vi "超标留样启动流程.vi"   [LabVIEW 2016, in "DR803M4.lvlib"]
uses:
  DR803M4.lvlib
  Global variable/input variable.vi
types:
  T1 = cluster{"远程留样":u16, "门禁标志":u16, "门禁密码":u32, "采样器进程":u16, "版本号":string, "启停":u16, "当前瓶号":u16, "采样模式选择":u16, "单次采样量":u16, "时间间隔":u16}
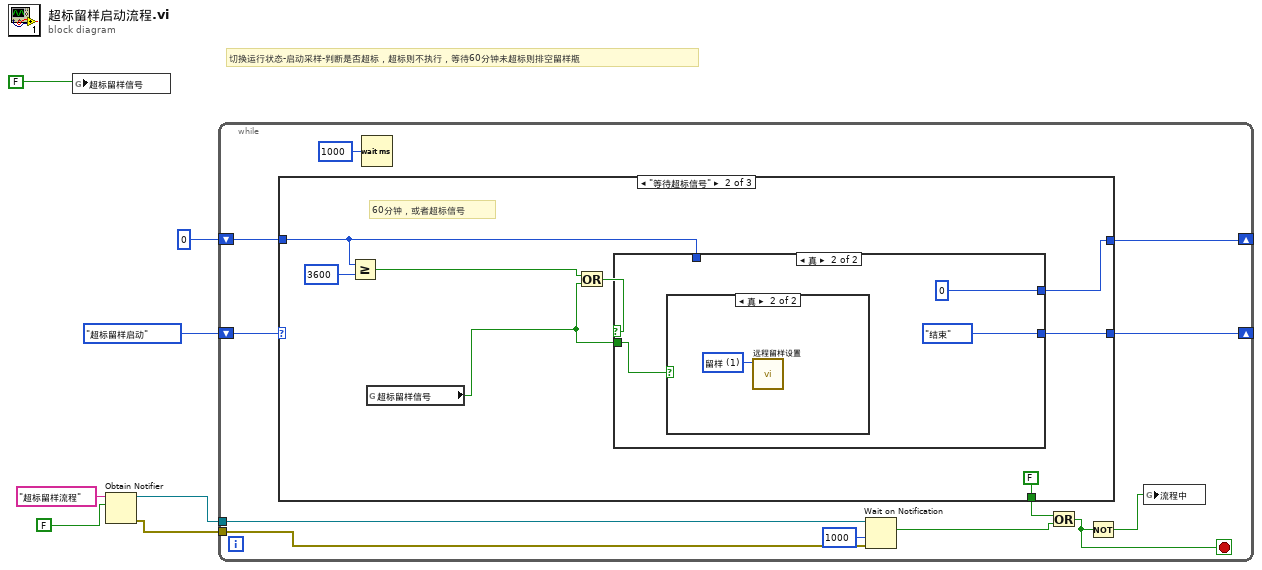
[diagram p0: block diagram]
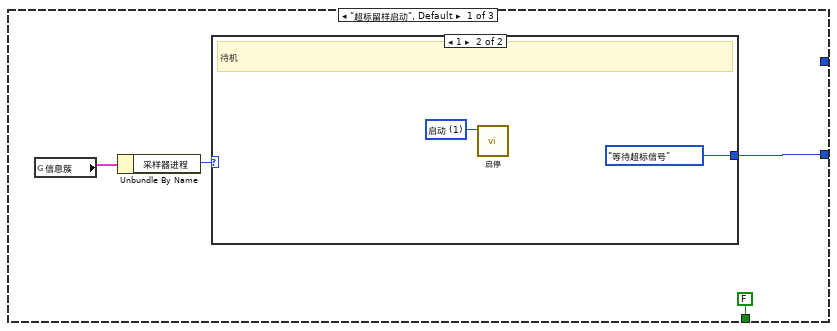
[diagram p2: hidden frame]
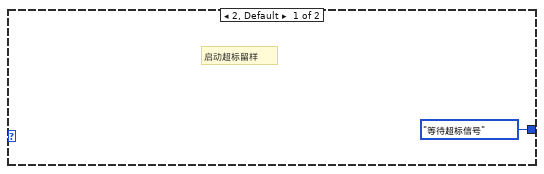
[diagram p3: hidden frame]
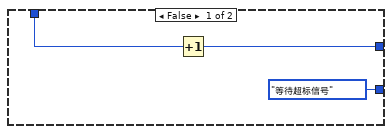
[diagram p4: hidden frame]
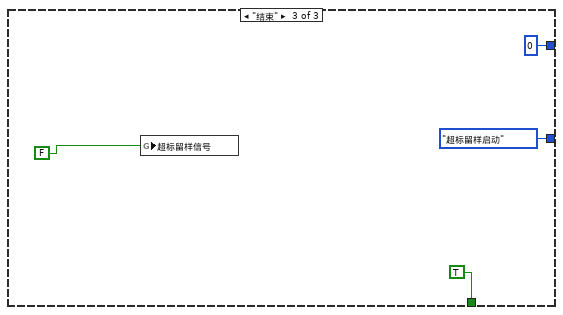
[diagram p6: hidden frame]
diagram:
  # "切换运行状态-启动采样-判断是否超标，超标则不执行，等待60分钟未超标则排空留样瓶"
  n1 = global write "input variable.vi" "超标留样信号"(FALSE ("采样完成")) -> ()
  n2 = Obtain Notifier(name (unnamed)="超标留样流程" ("名称（未命名）"), notification data type=FALSE ("采样完成")) -> (notifier out=w3:refnum<notifier>, error out=w2:errorcluster)  [unwired: 2 in, 1 out]
  n3 = while {
    shift-right: [w10] -> _
    shift-left: enum16{"超标留样启动", "等待超标信号", "结束"}."超标留样启动" -> [w19]
    shift-right: [w16] -> _
    shift-left: 0 -> [w17]
    tunnel: w3 -> [w15]
    tunnel: w2 -> [w14]
    stop <- w12 stop-if-true
    n4 = case shown="\"等待超标信号\"" w19 {
      tunnel: w17 -> [_ w30 _]
      tunnel: [_ w32 0] -> w16
      tunnel: [w21 w29 enum16{"超标留样启动", "等待超标信号", "结束"}."超标留样启动"] -> w10
      tunnel: [FALSE FALSE TRUE] -> w9
      frame "超标留样启动", Default {
        n5 = global read "input variable.vi" "信息簇"() -> (w23:T1)
        n6 = Unbundle By Name(w23) -> ("采样器进程"=w22:u16)
        n7 = case shown="1" w22 {
          tunnel: [enum16{"超标留样启动", "等待超标信号", "结束"}."等待超标信号" enum16{"超标留样启动", "等待超标信号", "结束"}."等待超标信号"] -> w21
          frame 2, Default {
            # "启动超标留样"
          }
          frame 1 {
            w25 = u16 1 items=["停止", "启动"] ("启停")
            # "待机"
            n8 = call "启停.vi"("启停"=w25) -> ()  [unwired: 10 in, 1 out]
          }
        }
      }
      frame "等待超标信号" {
        # "60分钟，或者超标信号"
        n9 = Greater Or Equal?(x=w30, y=3600) -> (x >= y?=w33:bool)
        n10 = global read "input variable.vi" "超标留样信号"() -> (w27:bool)
        n11 = Or(x=w33, y=w27) -> (x .or. y?=w31:bool)
        n12 = case shown="真" w31 {
          tunnel: [enum16{"超标留样启动", "等待超标信号", "结束"}."等待超标信号" enum16{"超标留样启动", "等待超标信号", "结束"}."结束"] -> w29
          tunnel: w30 -> [w37 _]
          tunnel: [w36 0] -> w32
          tunnel: w27 -> [_ w38]
          frame False {
            n13 = Increment(x=w37) -> (x+1=w36:i32)
          }
          frame True {
            n14 = case shown="真" w38 {
              frame False {
              }
              frame True {
                w41 = u16 1 items=["停止", "留样"] ("远程留样")
                n15 = call "远程留样设置.vi"("远程留样"=w41) -> ()  [unwired: 10 in, 1 out]
              }
            }
          }
        }
      }
      frame "结束" {
        n16 = global write "input variable.vi" "超标留样信号"(FALSE ("采样完成")) -> ()
      }
    }
    n17 = Wait (ms)(milliseconds to wait=u32 1000 ("等待时间（毫秒）")) -> ()  [unwired: 1 out]
    n18 = Wait on Notification(notifier=w15, timeout in ms (-1)=1000 ("超时毫秒(-1)"), error in (no error)=w14) -> (notification=w11:bool)  [unwired: 1 in, 3 out]
    n19 = Or(x=w9, y=w11) -> (x .or. y?=w12:bool)
    n20 = Not(x=w12) -> (.not. x?=w8:bool)
    n21 = global write "input variable.vi" "流程中"(w8) -> ()
  }
